vi "Simple Encoder.vi"(2 "Encoder Reset Value":i32, 5 "Encoder Reset":bool, 6 "DIO.1/QE.B":refnum<k21>, 8 "DIO.0/QE.A":refnum<k21>) -> (14 "RAW A/B":fxp<+,2,2> format="%02b", 17 "Counter":i32)   [LabVIEW 2018]
uses:
  <vilib>/rvi/eio/common/nirviEmuTemplateMethod_errors.vi
  <vilib>/eio/EIONode/EIONode.xnode
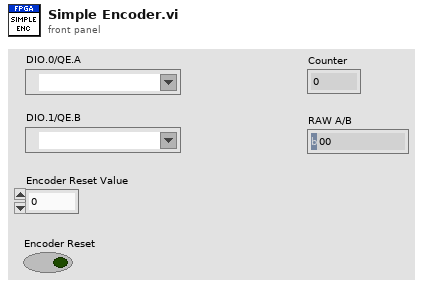
[diagram p1: front panel]
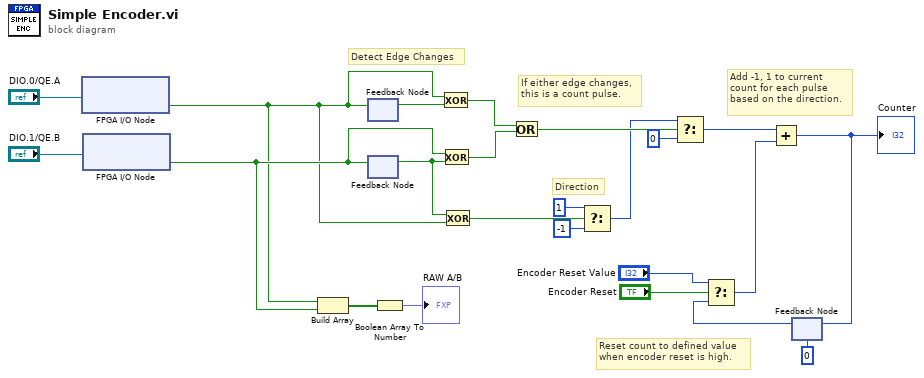
[diagram p0: block diagram]
diagram:
  # "Reset count to defined value\nwhen encoder reset is high."
  # "Add -1, 1 to current\ncount for each pulse\nbased on the direction."
  # "Direction"
  # "If either edge changes,\nthis is a count pulse."
  # "Detect Edge Changes"
  n1 = xnode "FPGA I/O Node"("FPGA I/O In"="DIO.0/QE.A") -> ("I/O Item"=w14:bool)  [unwired: 1 out]
  n2 = xnode "FPGA I/O Node"("FPGA I/O In"="DIO.1/QE.B") -> ("I/O Item"=w18:bool)  [unwired: 1 out]
  n3 = Build Array(w14, w18) -> (w23:bool[])
  n4 = feedback-in #1(w14) -> ()
  n5 = feedback #1() -> (w19:bool)  [unwired: 1 in]
  n6 = feedback #2() -> (w15:bool)  [unwired: 1 in]
  n7 = feedback-in #2(w18) -> ()
  n8 = Boolean Array To Number(Boolean array=w23) -> (number=→"RAW A/B":fxp<+,2,2>)
  n9 = Exclusive Or(1:w19, 2:w14) -> (0:w17:bool)
  n10 = Exclusive Or(1:w15, 2:w18) -> (0:w16:bool)
  n11 = Exclusive Or(1:w14, 2:w15) -> (0:w13:bool)
  n12 = Or(x=w17, y=w16) -> (x .or. y?=w10:bool)
  n13 = Select(t=1, s=w13, f=-1) -> (s? t:f=w9:i32)
  n14 = Select(t=w9, s=w10, f=0) -> (s? t:f=w7:i32)
  n15 = feedback #3(0) -> (w4:i32)
  n16 = Select(t="Encoder Reset Value", s="Encoder Reset", f=w4) -> (s? t:f=w2:i32)
  n17 = Add(x=w7, y=w2) -> (x+y=w6:i32)
  "Counter" <- w6
  n18 = feedback-in #3(w6) -> ()
